vi "Initialize_PIC.vi"(8 "error in (no error)":errorcluster, 10 "baud rate":u32=9600, 11 "Select Com Port":refnum<visa-resource-name>="COM1") -> (0 "error out":errorcluster, 3 "VISA resource name out":refnum<visa-resource-name>)   [LabVIEW 2017]
uses:
  <vilib>/Instr/_visa.llb/VISA Configure Serial Port (Instr).vi
panel:
  # "USB/VISA PIC Initialize"
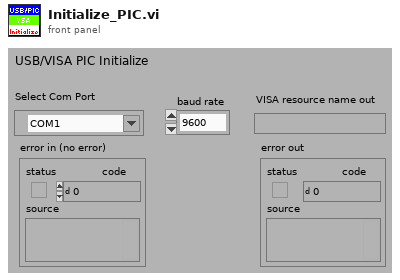
[diagram p1: front panel]
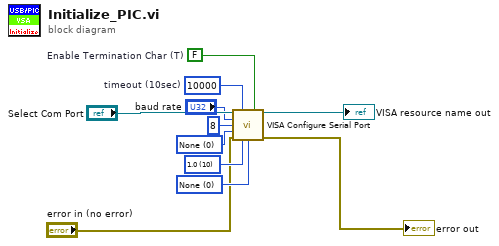
[diagram p0: block diagram]
diagram:
  w9 = u16 0 items=["None", "Odd", "Even", "Mark", "Space"] ("parity")
  w6 = u16 10 items=["1.0"=10, "1.5"=15, "2.0"=20] ("stop bits")
  w5 = u16 0 items=["None"=0, "XON/XOFF"=1, "RTS/CTS"=2, "DTR/DSR"=4] ("flow control")
  w7 = FALSE  # Enable Termination Char (T)
  w8 = u32 10000  # timeout (10sec)
  n1 = call-poly "VISA Configure Serial Port"("VISA resource name"="Select Com Port", "timeout (10sec)"=w8, "Enable Termination\nChar (T)"=w7, "baud rate (9600)"="baud rate", "data bits (8)"=u16 8 ("data bits"), "parity (0:none)"=w9, "error in (no error)"="error in (no error)", "stop bits (10: 1 bit)"=w6, "flow control (0:none)"=w5) -> ("VISA resource name out"=→"VISA resource name out":refnum<visa-resource-name>, "error out"=→"error out":errorcluster)  [unwired: 5 out]
